vi "PDF_Interface_PDF Protokoll EPA1065_550 Drift.vi"(8 "error in (no error)":errorcluster caption="Fehler (Eingang, kein Fehler)", 10 "Analysator":T1="FT-IR", 11 "Save PDF File Path":path) -> (0 "error out":errorcluster caption="Fehler (Ausgang)")   [LabVIEW 2020, in "EPA 1065.lvlib" / "Gas Analyzer Drift 1065-550.lvlib"]
uses:
  Gas Analyzer Drift 1065-550.lvlib
  Drifttabelle.ctl
  Seiten/System Einstellungen V2/Analysatoren.ctl
  Sprachverwaltung/FGV Aktion Tabelle zerlegen.ctl
  Seiten/FT-IR/FGV FT-IR Aktionen.ctl
  Chiller NO2 1065-376/Aktion FGV Drift Daten.ctl
  Seiten/System Einstellungen V2/Aktioen FGV System Konstanten.ctl
  PDF_Interface/PDF Protokoll Standard Kopf Optionen.ctl
  <vilib>/Simplicity AI/SAI_PDF_API/Classes/Context/Controls/SAI_PDF_PDF Details.ctl
  PDF_Interface/PDF Interface Helper/PDFContentType.ctl
  PDF_Interface/PDF Interface Helper/PDFTableContentType.ctl
  PDF_Interface/PDF Interface Helper/PDFResults.ctl
  PDF_Interface/PDF Interface Helper/PDFResultPictures.ctl
  PDF_Interface/PDF Interface Helper/PDFCommentPosition.ctl
  PDF_Interface/PDF Interface Helper/PDFPageBreak.ctl
  PDF_Interface/PDF Interface Helper/PDFTablePictures.ctl
  PDF_Interface/PDF Interface Helper/PDFBemerkung.ctl
  <vilib>/Simplicity AI/SAI_PDF_API/Classes/Context/Controls/SAI_PDF_Text Align.ctl
  <vilib>/Simplicity AI/SAI_PDF_API/Classes/Context/Controls/SAI_PDF_Font.ctl
  <vilib>/Simplicity AI/SAI_PDF_API/Classes/Context/Controls/SAI_PDF_Font Encoding.ctl
  Allgemein/allgemeine Sub-VIs.lvlib
  Seiten/FT-IR/FT-IR.lvlib
  Seiten/System Einstellungen V2/System Einstellungen V2.lvlib
  Sprachverwaltung/Sprachverwaltung.lvlib
  PDF_Interface/PDF Interface.lvlib
  PDF_Interface/PDF Interface Helper/PDF Interface Helper.lvlib
  <vilib>/Simplicity AI/SAI_PDF_API/Classes/Context/Context.lvclass
  Linearisierung V2/Protokoll/Protokoll.lvlib
panel:
  out "Drifttabelle":T2
  out "Versa Serial number:":string caption="Serial Nr.:"
  out "Anlage:":string caption="Device:"
  out "Methode (Recipe):":string
  out "Date & Time:":string caption="Datum & Uhrzeit:"
  out "Bearbeiter:":string
  # "Drift Test EPA § 1065.550"
  # "x"
  # "x"
  # "x"
  # "x"
  # "x"
  # "x"
  # "xidriftcorrected=xrefzero+(xrefspan-xrefzero)·2xi-(xprezero+xpostzero)(xprespan+xpostspan)-(xprezero+xpostzero)"
  # "Eq. 1065.672-1"
  # "xidriftcorrected = Konzentration um Drift korrigiert."
  # "xrefzero = Referenzkonzentration des Nullgases, die normalerweise Null ist, sofern nichts anderes bekannt ist."
  # "xrefspan = Referenzkonzentration des Kalibriergases."
  # "xprespan = Reaktion des Gasanalysators vor dem Testintervall auf die Kalibriergaskonzentration."
  # "xpostspan = Reaktion des Gasanalysators nach dem Testintervall auf die Spangaskonzentration."
  # "xi oder x = während des Tests aufgezeichnete Konzentration vor der Driftkorrektur."
  # "xprezero = Reaktion des Gasanalysators vor dem Testintervall auf die Nullgaskonzentration."
  # "xpostzero = Reaktion des Gasanalysators nach dem Testintervall auf die Nullgaskonzentration."
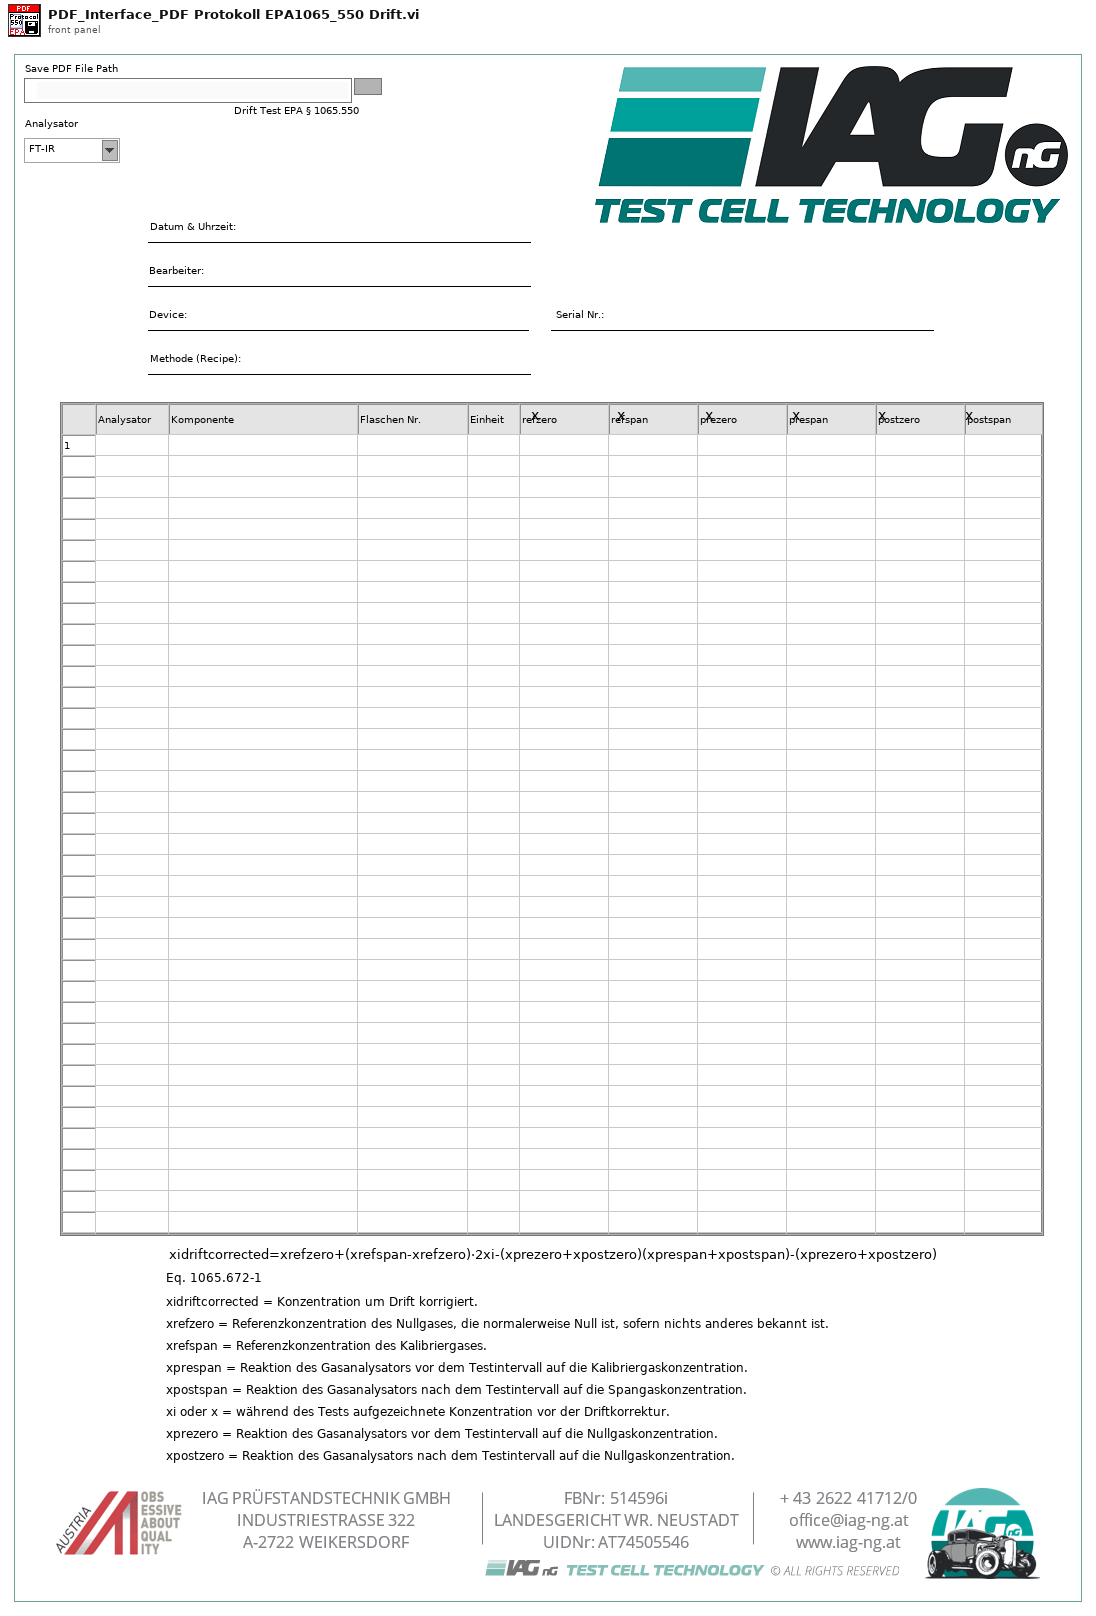
[diagram p1: front panel]
types:
  T1 = typedef "System Einstellungen V2.lvlib/Analysatoren.ctl" = string
  T2 = typedef "EPA 1065.lvlib/Gas Analyzer Drift 1065-550.lvlib/Drifttabelle.ctl" = string[][]
  T3 = typedef "Sprachverwaltung.lvlib/FGV Aktion Tabelle zerlegen.ctl" = enum16{"laden", "vereinzeln", "speichern"}
  T4 = typedef "PDF Interface.lvlib/PDF Protokoll Standard Kopf Optionen.ctl" = cluster{"Analysator":bool, "FT-IR Rezept":bool, "Gasteiler":bool, "Gas Komponente":bool, "Gas Flasche":bool, "LIN Protokoll":bool, "Operator":bool}
  T5 = typedef "System Einstellungen V2.lvlib/Aktioen FGV System Konstanten.ctl" = enum16{"lesen", "laden", "speichern", "Sprache"}
  T6 = typedef "EPA 1065.lvlib/Gas Analyzer Drift 1065-550.lvlib/Aktion FGV Drift Daten.ctl" = enum16{"lesen", "Konfig Daten", "PDF einstellen", "laden", "speichern", "Tabelle init", "Zeile Prüfen", "Info schreiben", "Span Einstellung", "Pre Werte schreiben", "Post Werte schreiben", "NB Pre Wert schreiben", "NB Post Wert schreiben", "Tabelle löschen"}
  T7 = typedef "FT-IR.lvlib/FGV FT-IR Aktionen.ctl" = enum16{"lesen", "NOG setzen", "NOS setzen", "Initialisieren", "speichern", "ALLES setzen", "FT-IR Spektrum loggen", "Komm Stoppen", "Spektrum LogKonfig"}
  T8 = typedef "PDF Interface.lvlib/PDF Interface Helper.lvlib/PDFBemerkung.ctl" = cluster{"Bemerkung Text":string, "Align (Left)":T9, "Add Line Feeds (F:No)":bool, "Font":T10}
  T9 = typedef "SAI_PDF_Toolkit.lvlib/Context.lvclass/SAI_PDF_Text Align.ctl" = i32
  T10 = typedef "SAI_PDF_Toolkit.lvlib/Context.lvclass/SAI_PDF_Font.ctl" = cluster{"Font":string, "Size":i32, "Colour":u32, "Bold":bool, "Italic":bool, "Underline":bool, "Strikethrough":bool, "Font Encoding":T11}
  T11 = typedef "SAI_PDF_Toolkit.lvlib/Context.lvclass/SAI_PDF_Font Encoding.ctl" = enum16{"Cp1252, WinANSI", "IdentityH", "IdentityV", "Cp1250", "Cp1257", "MacRoman"}
  T12 = typedef "PDF Interface.lvlib/PDF Interface Helper.lvlib/PDFTableContentType.ctl" = cluster{"TableHeader":string[], "Table":string[][], "Relative Column Widths (%)":sgl[], "Results":T13, "PositionBemerkung":T15, "PageBreak":T16, "TablePictures":T17, "Horizontal Align":i32}
  T13 = typedef "PDF Interface.lvlib/PDF Interface Helper.lvlib/PDFResults.ctl" = cluster{"Results":cluster{"Result Text":string, "Result":bool}[], "ResultPictures":T14, "use Pictures":bool, "Image Scale (%)":sgl, "Autoscale? (T)":bool, "Horizontal Align":i32, "Position":i32}
  T14 = typedef "PDF Interface.lvlib/PDF Interface Helper.lvlib/PDFResultPictures.ctl" = cluster{"Yes Ctl Refnum":refnum<vi>, "No Ctl Refnum":refnum<vi>}
  T15 = typedef "PDF Interface.lvlib/PDF Interface Helper.lvlib/PDFCommentPosition.ctl" = enum16{"before", "after"}
  T16 = typedef "PDF Interface.lvlib/PDF Interface Helper.lvlib/PDFPageBreak.ctl" = enum16{"none", "before", "after", "after comment"}
  T17 = typedef "PDF Interface.lvlib/PDF Interface Helper.lvlib/PDFTablePictures.ctl" = cluster{"Ctl Refnum In":refnum<vi>[], "RowOrColumn":enum16{"Row", "Column"}, "IndexToInsert":u16, "Image Scale (%)":sgl[], "Autoscale? (T)":bool[], "Horizontal Align":i32}
  T18 = typedef "PDF Interface.lvlib/PDF Interface Helper.lvlib/PDFContentType.ctl" = cluster{"Titel":string, "Header Table":string[][], "Table Array":T12[], "Bemerkungen":T8[]}
  T19 = typedef "SAI_PDF_Toolkit.lvlib/Context.lvclass/SAI_PDF_PDF Details.ctl" = cluster{"Title":string, "Subject":string, "Keywords":string, "Author":string, "Creator":string}
  T20 = cluster{"Header Footer Text Cluster":cluster{"Header Text":string, "Footer Text":string, "Time":string, "Page Number":string}, "PDF Details":T19}
  T21 = typedef "EPA 1065.lvlib/Gas Analyzer Drift 1065-550.lvlib/Konfig Daten Drift Verification.ctl" = cluster{"Bearbeiter:":string, "Pfad:":path, "Textname:":string, "CG Aufschaltzeit:":dbl, "N2 Aufschaltzeit:":dbl}
  T22 = cluster{"Modell":string, "ProjektNummer":string, "Software Version":string, "Seriennummer":string}
  T23 = cluster{"Header Size":i32, "Column Ratio left":sgl[]}
  T24 = typedef "String - Ausgabefeld.ctl" = string
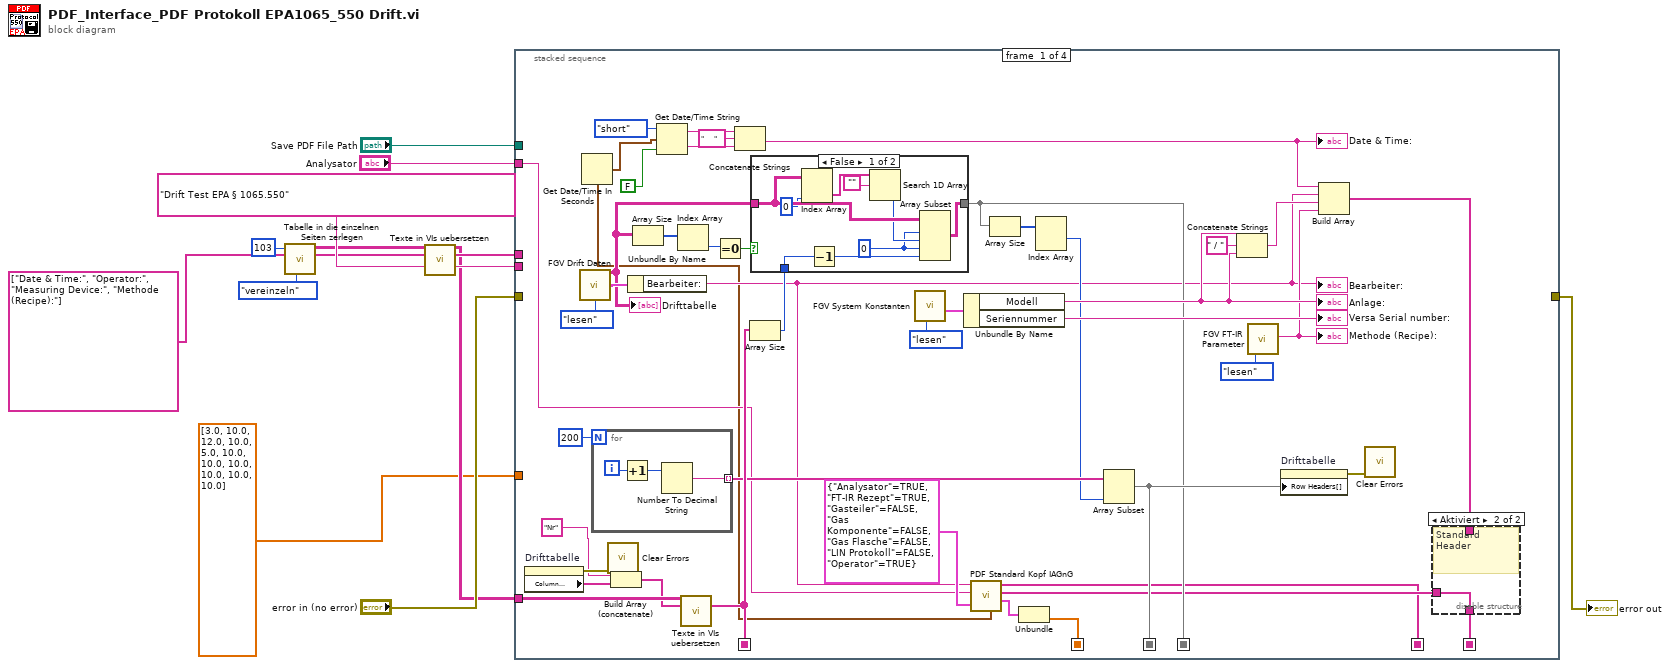
[diagram p0: block diagram]
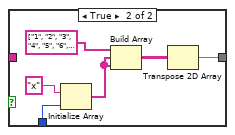
[diagram p3: hidden frame]
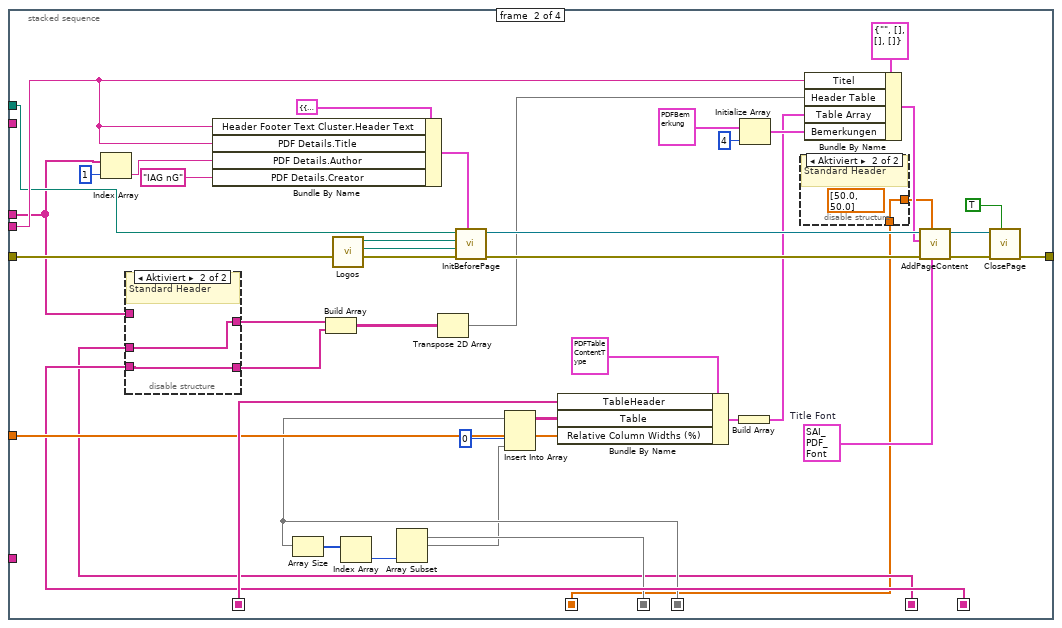
[diagram p4: hidden frame]
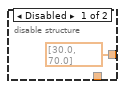
[diagram p5: hidden frame]
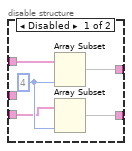
[diagram p6: hidden frame]
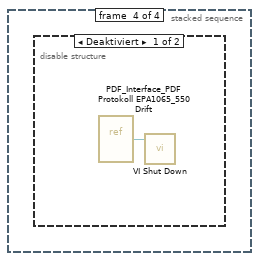
[diagram p8: hidden frame]
diagram:
  n1 = call "Tabelle in die einzelnen Seiten zerlegen.vi"("Aktion"=FGV_Aktion_Tabelle_zerlegen."vereinzeln", "Index (Seite)"=103) -> ("Sprachliste"=w10:string[][])  [unwired: 7 in, 2 out]
  n2 = call "Texte in VIs uebersetzen.vi"("Sprachliste"=w10, "String-Array zum Übersetzen"=string[] ["Date & Time:", "Operator:", "Measuring Device:", "Methode (Recipe):"], "String zum Übersetzen"="Drift Test EPA § 1065.550") -> ("Sprachliste out"=w4:string[][], "String-Array zum Übersetzen"=w8:string[], "String zum Übersetzen"=w7:string)  [unwired: 8 in, 2 out]
  n3 = stacked-sequence {
    seq-local: [w20 _ _ _] -> [_ w91 _ _]
    seq-local: [w26 _ _ _] -> [_ w87 _ _]
    seq-local: [w31 _ _ _] -> [_ w94 _ _]
    seq-local: [w27 _ _ _] -> [_ w88 _ _]
    seq-local: [w17 _ _ _] -> [_ w79 _ _]
    seq-local: [w14 _ _ _] -> [_ w78 _ _]
    tunnel: w8 -> [_ w92 _ _]
    tunnel: w7 -> [_ w97 _ _]
    tunnel: "Save PDF File Path" -> [_ w96 _ _]
    tunnel: "error in (no error)" -> [_ w95 _ _]
    tunnel: w4 -> [w34 _ _ _]
    tunnel: sgl[] [3.0, 10.0, 12.0, 10.0, 5.0, 10.0, 10.0, 10.0, 10.0, 10.0, 10.0] ("Relative Column Widths (%)") -> [_ w93 _ _]
    tunnel: [_ w83 _ _] -> w2
    tunnel: "Analysator" -> [w21 _ _ _]
    frame #0 {
      n4 = property on="Drifttabelle" class="Tbl (strikt)"() -> (error out=w35:errorcluster, "Column Headers[]"=w32:string[])  [unwired: 2 in, 1 out]
      n5 = call "FGV Drift Daten.vi"("Aktion"=Aktion_FGV_Drift_Daten."lesen") -> ("Drifttabelle"=w36:T2, "Drift Konfig Daten"=w50:T21)  [unwired: 7 in, 6 out]
      "Drifttabelle" <- w36
      n6 = Get Date/Time In Seconds() -> (seconds since 1Jan1904=w16:timestamp)
      n7 = for {
        N: 200 -> [_]
        tunnel: [w75] -> w30 mode=indexing
        i -> [w77]
        n8 = Increment(x=w77) -> (x+1=w76:i32)
        n9 = Number To Decimal String(number=w76) -> (decimal integer string=w75:string)  [unwired: 1 in]
      }
      n10 = call <vilib>:"Clear Errors.vi"("error in (no error)"=w35) -> ()  [unwired: 5 in, 2 out]
      n11 = Build Array (concatenate)("Nr", w32) -> (w25:string[])
      n12 = Unbundle By Name(w50) -> ("Bearbeiter:"=w22:string)
      "Bearbeiter:" <- w22
      n13 = Array Size(array=w36) -> (size(s)=w39:i32[])
      n14 = Get Date/Time String(date format (0)=enum16{"short", "long", "abbreviated"}."short" ("Datumsformat (0)"), seconds (now)=w16, want seconds? (F)=FALSE ("Angabe von Sekunden? (F)")) -> (date string=w57:string, time string=w56:string)
      n15 = Index Array(array=w39) -> (element=w38:i32)  [unwired: 1 in]
      n16 = call "Texte in VIs uebersetzen.vi"("Sprachliste"=w34, "String-Array zum Übersetzen"=w25) -> ("String-Array zum Übersetzen"=w31:string[])  [unwired: 9 in, 4 out]
      n17 = Equal To 0?(x=w38) -> (x = 0?=w37:bool)
      n18 = Concatenate Strings(w57, "     " ("String"), w56) -> (w42:string)
      "Date & Time:" <- w42
      n19 = Array Size(array=w31) -> (size(s)=w33:i32)
      n20 = case shown="False" w37 {
        tunnel: [w63 w70] -> w26
        tunnel: w36 -> [w68 _]
        tunnel: w33 -> [w60 w69]
        frame False {
          w64 = 0 ("Index")
          n21 = Index Array(array=w68, index (col)=0 ("Index")) -> (element=w67:string[])  [unwired: 1 in]
          n22 = Decrement(x=w60) -> (x-1=w61:i32)
          n23 = Search 1D Array(1D array=w67, element="") -> (index of element=w65:i32)  [unwired: 1 in]
          n24 = Array Subset(array=w68, index (row)=w64, length (row)=w65, index (col)=w64, length (col)=w61) -> (w63:T2)
        }
        frame True {
          n25 = Initialize Array("x", w69) -> (w72:string[])
          n26 = Build Array(string[] ["1", "2", "3", "4", "5", "6", "7"], w72, w72) -> (w71:string[][])
          n27 = Transpose 2D Array(2D array=w71) -> (transposed array=w70:string[][])
        }
      }
      n28 = call "FGV System Konstanten.vi"("Aktionen"=Aktioen_FGV_System_Konstanten."lesen") -> ("Cluster out"=w46:T22)  [unwired: 6 in, 4 out]
      n29 = Unbundle By Name(w46) -> ("Modell"=w43:string, "Seriennummer"=→"Versa Serial number:":string)
      "Anlage:" <- w43
      n30 = call "PDF Standard Kopf IAGnG.vi"("Zeitstempel"=w16, "Oprtionen Cluster"=T4 {"Analysator"=TRUE, "FT-IR Rezept"=TRUE, "Gasteiler"=FALSE, "Gas Komponente"=FALSE, "Gas Flasche"=FALSE, "LIN Protokoll"=FALSE, "Operator"=TRUE}, "Analysator"=w21, "Bearbeiter/in"=w22) -> ("Size Cluster"=w15:T23, "Header Values"=w18:T24[], "Header Labels"=w17:string[])  [unwired: 4 in, 1 out]
      n31 = Array Size(array=w26) -> (size(s)=w29:i32[])
      n32 = Unbundle(w15) -> ("Column Ratio left"=w14:sgl[])  [unwired: 1 out]
      n33 = Index Array(array=w29) -> (element #1=w28:i32)  [unwired: 2 in, 1 out]
      n34 = Array Subset(array=w30, length=w28) -> (w27:string[])  [unwired: 1 in]
      n35 = Concatenate Strings(w43, " / " ("String"), w43) -> (w41:string)
      n36 = call "FGV FT-IR Parameter.vi"("Aktion"=FGV_FT-IR_Aktionen."lesen") -> ("Current Recipe"=w40:string)  [unwired: 11 in, 7 out]
      "Methode (Recipe):" <- w40
      n37 = property on="Drifttabelle" class="Tbl (strikt)"("Row Headers[]"=w27) -> (error out=w47:errorcluster)  [unwired: 2 in, 1 out]
      n38 = Build Array(w42, w22, w41, w40) -> (w19:string[])
      n39 = call <vilib>:"Clear Errors.vi"("error in (no error)"=w47) -> ()  [unwired: 5 in, 2 out]
      n40 = disable-structure shown="Aktiviert" {
        disable-tunnel: [w58 w59] -> w20
        disable-tunnel: w19 -> [w58 _]
        disable-tunnel: w18 -> [_ w59]
        frame Disabled {
        }
        frame Enabled {
          # "Standard Header"
        }
      }
    }
    frame #1 {
      w101 = T10 {"Font"="Arial", "Size"=26, "Colour"=0, "Bold"=TRUE, "Italic"=FALSE, "Underline"=TRUE, "Strikethrough"=FALSE, "Font Encoding"=enum."Cp1252, WinANSI"}  # Title Font
      n41 = Index Array(array=w92, index=1 ("Index")) -> (element=w98:string)
      n42 = disable-structure shown="Aktiviert" {
        disable-tunnel: [w127 w128] -> w109
        disable-tunnel: [w126 w129] -> w108
        disable-tunnel: w92 -> [w124 _]
        disable-tunnel: w91 -> [w123 w129]
        disable-tunnel: w79 -> [_ w128]
        frame Disabled {
          w125 = 4 ("Länge")
          n43 = Array Subset(array=w124, length=w125) -> (w127:string[])  [unwired: 1 in]
          n44 = Array Subset(array=w123, length=w125) -> (w126:T24[])  [unwired: 1 in]
        }
        frame Enabled {
          # "Standard Header"
        }
      }
      n45 = Bundle By Name(cluster=T20 {"Header Footer Text Cluster"={"Header Text"="Protokoll XYZ", "Footer Text"="IAG nG", "Time"="<TIMESTAMP yyyy-MM-dd>", "Page Number"="Page <P> of <PT>"}, "PDF Details"={"Title"="Test PDF", "Subject"="Versa Tabasco", "Keywords"="", "Author"="RIW", "Creator"="IAG"}} ("Info"), "Header Footer Text Cluster.Header Text"=w97, "PDF Details.Title"=w97, "PDF Details.Author"=w98, "PDF Details.Creator"="IAG nG") -> (w111:T20)
      n46 = Array Size(array=w87) -> (size(s)=w86:i32[])
      n47 = Build Array(w109, w108) -> (w107:T24[][])
      n48 = call "Logos.vi"() -> ("Footer Image File Path"=w119:path, "Header Image File Path"=w120:path)  [unwired: 8 in, 2 out]
      n49 = Index Array(array=w86) -> (element=w85:i32)  [unwired: 1 in]
      n50 = Array Subset(array=w88, length=w85) -> (w84:string[])  [unwired: 1 in]
      n51 = Transpose 2D Array(2D array=w107) -> (transposed array=w104:T24[][])
      n52 = call "InitBeforePage.vi"("Info"=w111, "Fehler (Eingang, kein Fehler)"=w95, "Footer Image File Path"=w119, "Header Image File Path"=w120, "Path (Dialog if Empty)"=w96) -> ("Fehler (Ausgang)"=w118:errorcluster, "Context (Ausgang)"=w117:refnum<class "Context.lvclass">)  [unwired: 5 in]
      n53 = Insert Into Array(array=w87, index (col)=0 ("Deaktivierter Index (Spalte)"), new element=w84) -> (w90:string[][])  [unwired: 1 in]
      n54 = Bundle By Name(cluster=T12 {"TableHeader"=[], "Table"=[], "Relative Column Widths (%)"=[], "Results"={"Results"=[], "ResultPictures"={"Yes Ctl Refnum"=refnum, "No Ctl Refnum"=refnum}, "use Pictures"=FALSE, "Image Scale (%)"=0.0, "Autoscale? (T)"=FALSE, "Horizontal Align"=0, "Position"=0}, "PositionBemerkung"=enum."before", "PageBreak"=enum."none", "TablePictures"={"Ctl Refnum In"=[], "RowOrColumn"=enum."Row", "IndexToInsert"=0, "Image Scale (%)"=[], "Autoscale? (T)"=[], "Horizontal Align"=0}, "Horizontal Align"=0} ("Table Content"), "TableHeader"=w94, "Table"=w90, "Relative Column Widths (%)"=w93) -> (w100:T12)
      n55 = Build Array(w100) -> (w82:T12[])
      n56 = Initialize Array(T8 {"Bemerkung Text"="", "Align (Left)"=0, "Add Line Feeds (F:No)"=FALSE, "Font"={"Font"="Arial", "Size"=10, "Colour"=0, "Bold"=FALSE, "Italic"=FALSE, "Underline"=FALSE, "Strikethrough"=FALSE, "Font Encoding"=enum."Cp1252, WinANSI"}} ("Bemerkung"), 4 ("Dimensionsgröße")) -> (w103:T8[])
      n57 = disable-structure shown="Aktiviert" {
        disable-tunnel: [sgl[] [30.0, 70.0] ("Column Ratio left") w122] -> w105
        disable-tunnel: w78 -> [_ w122]
        frame Disabled {
        }
        frame Enabled {
          (unwired) sgl[] [50.0, 50.0] ("Column Ratio left")
          # "Standard Header"
        }
      }
      n58 = Bundle By Name(cluster=T18 {"Titel"="", "Header Table"=[], "Table Array"=[], "Bemerkungen"=[]} ("Content"), "Titel"=w97, "Header Table"=w104, "Table Array"=w82, "Bemerkungen"=w103) -> (w106:T18)
      n59 = call "AddPageContent.vi"("Title Font"=w101, "Column Ratio left"=w105, "error in"=w118, "Content"=w106, "Context (Eingang)"=w117) -> ("error out"=w116:errorcluster, "Context (Ausgang)"=w115:refnum<class "Context.lvclass">)  [unwired: 5 in]
      n60 = call "ClosePage.vi"("popup viewer"=TRUE, "Fehler (Eingang, kein Fehler)"=w116, "Context (Eingang)"=w115) -> ("Fehler (Ausgang)"=w83:errorcluster)  [unwired: 8 in]
    }
    frame #2 {
    }
    frame #3 {
      n61 = disable-structure shown="Deaktiviert" {
        frame Disabled {
          n62 = vi-ref "PDF_Interface_PDF Protokoll EPA1065_550 Drift.vi"() -> (w130:refnum<vi>)
          n63 = call "VI Shut Down.vi"("VI Referenz"=w130) -> ()  [unwired: 11 in]
        }
        frame Enabled {
        }
      }
    }
  }
  "error out" <- w2
